vi "Main Engine Sync&Async DynData  File Read.vi"(8 "error in":errorcluster, 10 "Column":i32, 11 "File Name":string) -> (0 "error out":errorcluster, 3 "File DynData":sgl[](array[numeric]))   [LabVIEW 2021]
doc: "All Rights Reserved © 2017 SyncSols"
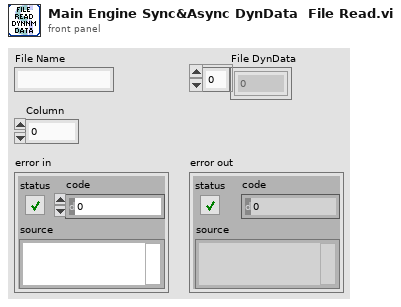
[diagram p1: front panel]
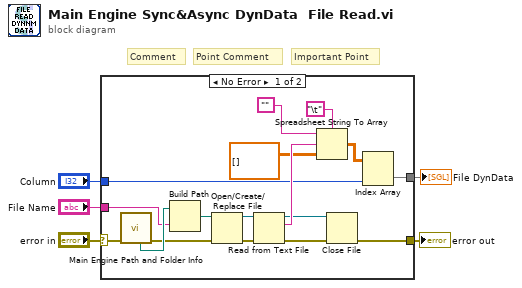
[diagram p0: block diagram]
diagram:
  # "Important Point"
  # "Point Comment"
  # "Comment"
  n1 = case shown="No Error" "error in" {
    selector: "error in" -> [w22 w23]
    tunnel: [w9 w23] -> w5
    tunnel: "File Name" -> [w20 _]
    tunnel: "Column" -> [w14 _]
    tunnel: [w7 _] -> w1
    frame No Error {
      n2 = call "Main Engine Path and Folder Info.vi"("error in"=w22) -> ("error out"=w19:errorcluster, "DynData File"=w21:path)  [unwired: 4 in, 5 out]
      n3 = Build Path(base path=w21, name or relative path=w20) -> (appended path=w18:path)
      n4 = Open/Create/Replace File(file path (use dialog)=w18, error in=w19) -> (refnum out=w16:refnum<file>, error out=w17:errorcluster)  [unwired: 4 in, 1 out]
      n5 = Read from Text File(file (use dialog)=w16, error in=w17) -> (refnum out=w11:refnum<file>, text=w15:string, error out=w10:errorcluster)  [unwired: 2 in, 1 out]
      n6 = Spreadsheet String To Array(delimiter (Tab)="\t", format string="", spreadsheet string=w15, array type (2D Dbl)=sgl[][] []) -> (array=w12:sgl[][])
      n7 = Close File(refnum=w11, error in=w10) -> (error out=w9:errorcluster)  [unwired: 1 out]
      n8 = Index Array(array=w12, index (col)=w14) -> (element=w7:sgl[])  [unwired: 1 in]
    }
    frame Error {
    }
  }
  "error out" <- w5
  "File DynData" <- w1
